vi "calculate_frames_per_second_count_dropped_frames.vi"(9 "Reset":bool, 10 "Update Interval (ms)":u32=1000, 11 "Buffer Number":u32) -> (1 "Missed Frames":dbl, 2 "Processed Frames/s":dbl, 3 "Acquired Frames/s":dbl)   [LabVIEW 2019]
doc: "Calculate the frame rate from within a loop. Frame rate is averaged over the specified update interval. The default update interval is 1000ms."
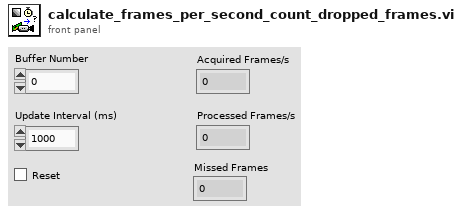
[diagram p1: front panel]
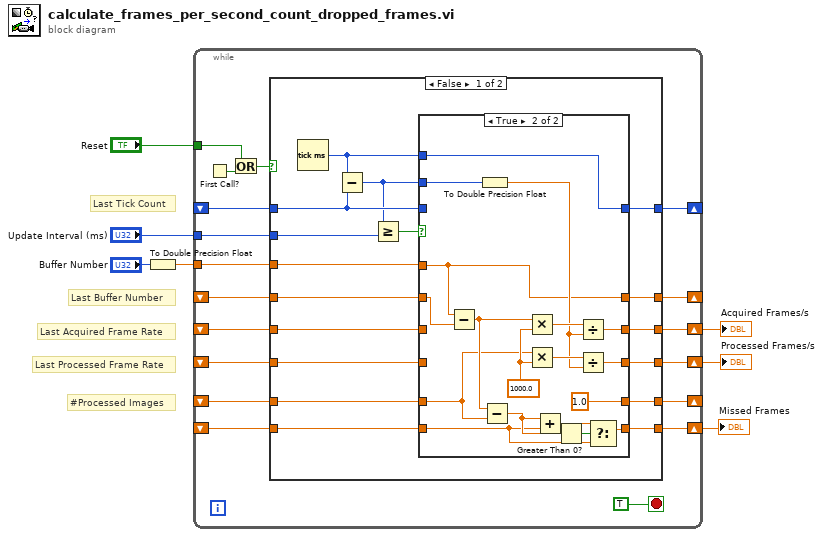
[diagram p0: block diagram]
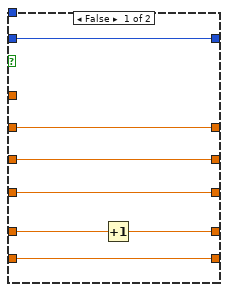
[diagram p2: hidden frame]
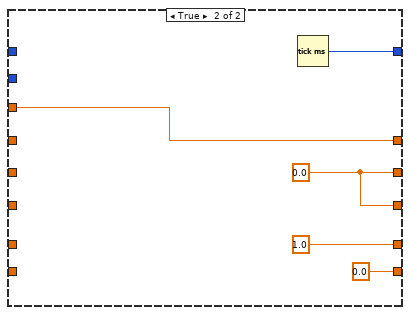
[diagram p3: hidden frame]
diagram:
  # "Last Processed Frame Rate"
  # "#Processed Images"
  # "Last Buffer Number"
  # "Last Acquired Frame Rate"
  # "Last Tick Count"
  n1 = To Double Precision Float(number="Buffer Number") -> (double precision float=w2:dbl)
  n2 = while {
    shift-right: [w24] -> _
    shift-left: _ -> [w23]
    shift-right: [w21] -> _
    shift-left: _ -> [w22]
    shift-right: [w20] -> w7
    shift-left: _ -> [w19]
    shift-right: [w18] -> _
    shift-left: _ -> [w17]
    shift-right: [w16] -> w6
    shift-left: _ -> [w15]
    tunnel: "Update Interval (ms)" -> [w14]
    tunnel: w2 -> [w10]
    tunnel: "Reset" -> [w9]
    shift-right: [w13] -> w4
    shift-left: _ -> [w8]
    stop <- TRUE stop-if-true
    n3 = First Call?() -> (First Call?: T/F=w12:bool)
    n4 = Or(x=w9, y=w12) -> (x .or. y?=w11:bool)
    n5 = case shown="False" w11 {
      tunnel: [w40 w72] -> w24
      tunnel: w23 -> [w41 _]
      tunnel: w22 -> [w39 _]
      tunnel: [w38 w71] -> w21
      tunnel: [w35 w69] -> w20
      tunnel: w19 -> [w34 _]
      tunnel: w10 -> [w33 w71]
      tunnel: [w31 1.0 ("buffer number")] -> w18
      tunnel: w17 -> [w32 _]
      tunnel: [w30 w69] -> w16
      tunnel: w15 -> [w29 _]
      tunnel: w14 -> [w28 _]
      tunnel: [w27 0.0] -> w13
      tunnel: w8 -> [w26 _]
      frame False {
        n6 = Tick Count (ms)() -> (millisecond timer value=w37:u32)
        n7 = Subtract(x=w37, y=w41) -> (x-y=w36:u32)
        n8 = Greater Or Equal?(x=w36, y=w28) -> (x >= y?=w42:bool)
        n9 = case shown="True" w42 {
          tunnel: w41 -> [w49 _]
          tunnel: [w49 w67] -> w40
          tunnel: w39 -> [w47 w64]
          tunnel: [w47 w57] -> w38
          tunnel: w37 -> [_ w67]
          tunnel: w36 -> [_ w61]
          tunnel: [w48 w65] -> w35
          tunnel: w34 -> [w48 _]
          tunnel: w33 -> [_ w57]
          tunnel: w32 -> [w46 w56]
          tunnel: [w45 1.0] -> w31
          tunnel: [w44 w60] -> w30
          tunnel: w29 -> [w44 _]
          tunnel: [w43 w51] -> w27
          tunnel: w26 -> [w43 w50]
          frame False {
            n10 = Increment(x=w46) -> (x+1=w45:dbl)
          }
          frame True {
            w63 = 1000.0 ("y")
            n11 = Subtract(x=w57, y=w64) -> (x-y=w58:dbl)
            n12 = To Double Precision Float(number=w61) -> (double precision float=w59:dbl)
            n13 = Subtract(x=w58, y=w56) -> (x-y=w55:dbl)
            n14 = Multiply(x=w58, y=w63) -> (x*y=w66:dbl)
            n15 = Multiply(x=w56, y=w63) -> (x*y=w62:dbl)
            n16 = Add(x=w55, y=w50) -> (x+y=w52:dbl)
            n17 = Greater Than 0?(x=w55) -> (x > 0?=w53:bool)
            n18 = Divide(x=w66, y=w59) -> (x/y=w65:dbl)
            n19 = Divide(x=w62, y=w59) -> (x/y=w60:dbl)
            n20 = Select(t=w52, s=w53, f=w50) -> (s? t:f=w51:dbl)
          }
        }
      }
      frame True {
        w69 = 0.0
        n21 = Tick Count (ms)() -> (millisecond timer value=w72:u32)
      }
    }
  }
  "Acquired Frames/s" <- w7
  "Processed Frames/s" <- w6
  "Missed Frames" <- w4
